vi "QCP_Set.vi"   [LabVIEW 2016]
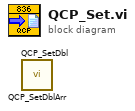
[diagram p0: block diagram]
diagram:
  n1 = call <userlib>:"QCP_SetDblArr.vi"() -> ()  [unwired: 10 in, 2 out]
  n2 = call <userlib>:"QCP_SetDbl.vi"() -> ()  [unwired: 10 in, 2 out]
